vi "Not a Refnum.vi"(4 "Priority Queue.lvclass":T1) -> (1 "NaN/Path/Refnum?":bool)   [LabVIEW 2017, in "Communicable State Machine.lvlib"]
doc: "### Not a Refnum.vi\n\n-- <b>Controls</b> --\n- <b>Priority Queue.lvclass</b>:\n\n-- <b>Indicators</b> --\n- <b>NaN/Path/Refnum?</b>:"
uses:
  Communicable State Machine.lvlib
  Priority Queue.ctl
  Typedef/_Cross CSM State Data.ctl
  Typedef/_CSM_MSG_TYPE.ctl
  Typedef/_Cross CSM State Response.ctl
  Typedef/_CSM_Response Source Message.ctl
  def-Data(LowPRI-Q).ctl
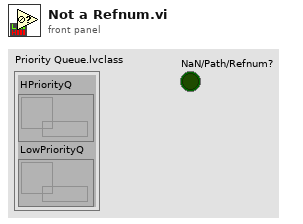
[diagram p1: front panel]
types:
  T1 = typedef "Communicable State Machine.lvlib/Priority Queue.ctl" = cluster{"HPriorityQ":refnum<queue>, "LowPriorityQ":refnum<queue>}
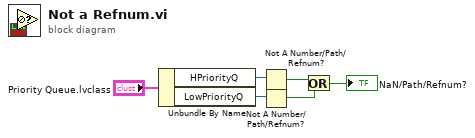
[diagram p0: block diagram]
diagram:
  n1 = Unbundle By Name("Priority Queue.lvclass") -> ("HPriorityQ"=w5:refnum<queue>, "LowPriorityQ"=w4:refnum<queue>)
  n2 = Not A Number/Path/Refnum?(number/path/refnum=w5) -> (NaN/Path/Refnum?=w3:bool)
  n3 = Not A Number/Path/Refnum?(number/path/refnum=w4) -> (NaN/Path/Refnum?=w2:bool)
  n4 = Or(x=w3, y=w2) -> (x .or. y?=→"NaN/Path/Refnum?":bool)
